vi "LinxDigitalWrite.vi"(8 "Error In":errorcluster, 9 "Values":bool[](array[boolean]), 10 "Channels":u8[](array[numeric]), 11 "LINX Resource":T1) -> (0 "Error Out":errorcluster, 3 "LINX Resource":T1)   [LabVIEW 2020, in "LMH-LINX.lvlib" / "Local IO.lvlib"]
uses:
  Local IO.lvlib
  Type Defs/LINX Ref.ctl
  Type Defs/Platform.ctl
  Device/Type Defs/LINX Device Config.ctl
  Type Defs/Interface.ctl
  Device/Type Defs/TCP Config.ctl
  Device/Type Defs/Channels.ctl
  <vilib>/MakerHub/LINX/Resources/liblinxdevice.dll
  LMH-LINX.lvlib
  Device/Device.lvlib
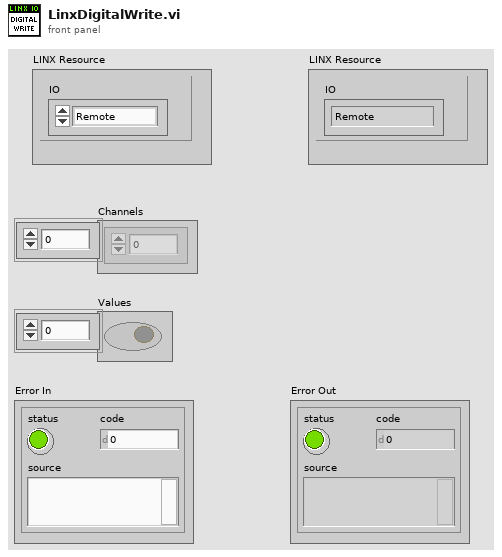
[diagram p1: front panel]
types:
  T1 = typedef "LMH-LINX.lvlib/LINX Ref.ctl" = cluster{"IO":T2, "LINX Device Config":T3}
  T2 = typedef "LMH-LINX.lvlib/Platform.ctl" = enum16{"Remote", "Local"}
  T3 = typedef "Device.lvlib/LINX Device Config.ctl" = cluster{"Interface":T4, "COM Port":refnum<visa-resource-name>, "TCP Configuration":T5, "Device Family":u8, "Device ID":u8, "Device Name":string, "TCP Ref":refnum<k5>, "Channels":T6}
  T4 = typedef "LMH-LINX.lvlib/Interface.ctl" = enum16{"Serial", "TCP"}
  T5 = typedef "Device.lvlib/TCP Config.ctl" = cluster{"IP Address":string, "Port":u16}
  T6 = typedef "LMH-LINX.lvlib/Channels.ctl" = cluster{"DI":u8[], "DO":u8[], "AI":u8[], "AO":u8[], "PWM":u8[], "QE":u8[], "UART":u8[], "I2C 2":u8[], "SPI":u8[], "CAN":u8[], "Servo":u8[], "AI Ref (V)":dbl, "AI Resolution (Bits)":u8, "AO Ref (V)":dbl, "AO Resolution (Bits)":u8}
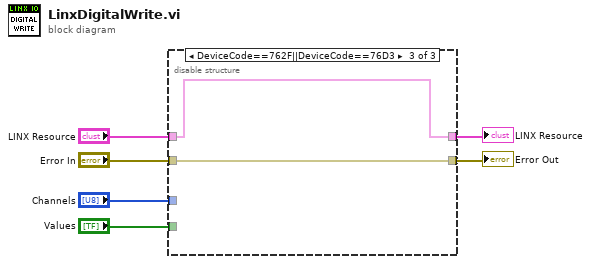
[diagram p0: block diagram]
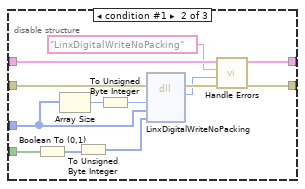
[diagram p3: hidden frame]
diagram:
  n1 = disable-structure shown="DeviceCode==762F||DeviceCode==76D3" {
    disable-tunnel: "LINX Resource" -> [w8 w11 w22]
    disable-tunnel: "Error In" -> [w7 w21 w23]
    disable-tunnel: [w7 w13 w23] -> w4
    disable-tunnel: [w8 w12 w22] -> w3
    disable-tunnel: "Channels" -> [_ w18 _]
    disable-tunnel: "Values" -> [_ w17 _]
    frame condition #0 (active) {
    }
    frame condition #1 {
      n2 = Boolean To (0,1)(Boolean=w17) -> (0, 1=w16:i16[])
      n3 = Array Size(array=w18) -> (size(s)=w20:i32)
      n4 = To Unsigned Byte Integer(number=w16) -> (unsigned 8bit integer=w15:u8[])
      n5 = To Unsigned Byte Integer(number=w20) -> (unsigned 8bit integer=w19:u8)
      n6 = dll-call lib="C:/Program Files (x86)/National Instruments/LabVIEW 2020/vi.lib/MakerHub/LINX/Resources/liblinxdevice.*" fn="LinxDigitalWriteNoPacking"(error in=w21, "numChans"=w19, "channels"=w18, "values"=w15) -> (error out=w14:errorcluster, "LinxStatus"=w9:i32)  [unwired: 5 in, 1 out]
      n7 = call "Handle Errors.vi"("Error In"=w14, "LinxStatus"=w9, "Function Name"="LinxDigitalWriteNoPacking", "LINX Resource"=w11) -> ("Error Out"=w13:errorcluster, "LINX Resource"=w12:T1)  [unwired: 6 in]
    }
    frame condition #2 {
    }
  }
  "Error Out" <- w4
  "LINX Resource" <- w3
